vi "LeCroy Wave Series Acquire and Read MyMeasurements.vi"() -> ()   [LabVIEW 2013]
doc: "This example shows how to use autosetup and acquire a waveform on a single channel."
uses:
  <instrlib>/LeCroy Wave Series/Public/Data/Read Waveform Measurement (Px).vi
  <instrlib>/LeCroy Wave Series/LeCroy Wave Series.lvlib
panel:
  out "Status":string
  out "Value":dbl format="%#_6p"
  in  "Parameter (0: P1)":u16(ring) items=["P1", "P2", "P3", "P4", "P5", "P6", "P7", "P8"]
  in  "VISA resource name":refnum<visa-resource-name>
  in  "Timeout (10000 ms)":u32=10000
  # "(c) 2008 - 2012 NATIONAL INSTRUMENTS.  ALL RIGHTS RESERVED."
  # "Directions:\n\n1. Setup the scope to be able to successfully single trigger on a signal applied to the channel selected in the \"Source\" control.\n\n2. On this front panel, enter the VISA Resource name for your scope. (e.g. VICP::123.45.67.8 for TCP/IP, GPIB::5::INSTR for GPIB). Modify the timeout if necessary.\n\n3. Select a parameter to read back\n\n4. Run the VI to trigger the scope and to read back the measurement result."
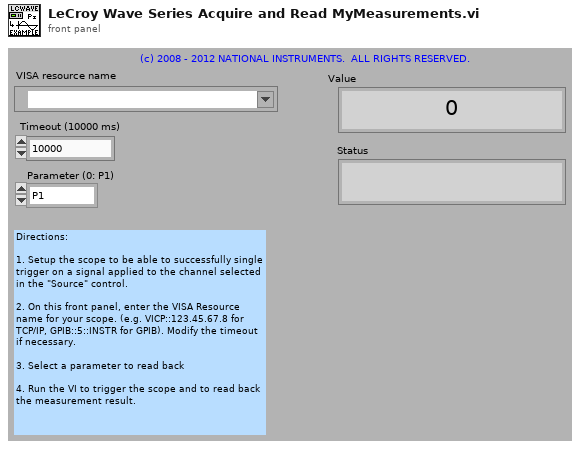
[diagram p1: front panel]
types:
  T1 = enum16{"MyMeasure", "Standard Vertical", "Standard Horizontal"}
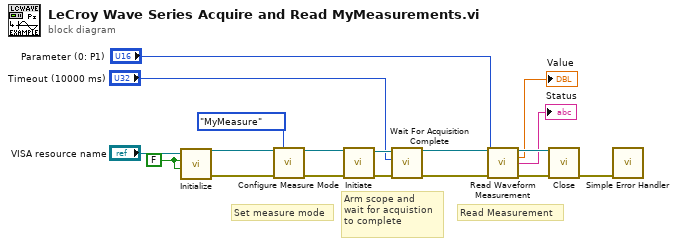
[diagram p0: block diagram]
diagram:
  w14 = FALSE ("ID Query? (T: Yes)")
  # "Arm scope and \nwait for acquistion\nto complete"
  # "Set measure mode"
  # "Read Measurement"
  n1 = call <instrlib>:"Initialize.vi"("Reset? (T: Yes)"=w14, "ID Query? (T: Yes)"=w14, "VISA resource name"="VISA resource name") -> ("error out"=w11:errorcluster, "VISA resource name out"=w13:refnum<visa-resource-name>)  [unwired: 7 in]
  n2 = call <instrlib>:"Configure Measure Mode.vi"("VISA resource name"=w13, "MeasureMode (0=MyMeasure)"=T1."MyMeasure", "error in (no error)"=w11) -> ("VISA resource name out"=w10:refnum<visa-resource-name>, "error out"=w9:errorcluster)  [unwired: 11 in]
  n3 = call <instrlib>:"Initiate.vi"("error in (no error)"=w9, "VISA resource name"=w10) -> ("error out"=w7:errorcluster, "VISA resource name out"=w8:refnum<visa-resource-name>)  [unwired: 8 in]
  n4 = call <instrlib>:"Wait For Acquisition Complete.vi"("error in (no error)"=w7, "Timeout (10000 ms)"="Timeout (10000 ms)", "VISA resource name"=w8) -> ("error out"=w6:errorcluster, "VISA resource name out"=w5:refnum<visa-resource-name>)  [unwired: 6 in, 1 out]
  n5 = call-poly <instrlib>:"Read Waveform Measurement.vi"("VISA resource name"=w5, "Parameter (0: P1)"="Parameter (0: P1)", "error in (no error)"=w6) -> ("VISA resource name out"=w17:refnum<visa-resource-name>, "Value"=→"Value":dbl, "Status"=→"Status":string, "error out"=w16:errorcluster)  [unwired: 9 in]
  n6 = call <instrlib>:"Close.vi"("error in (no error)"=w16, "VISA resource name"=w17) -> ("error out"=w18:errorcluster)  [unwired: 9 in]
  n7 = call <vilib>:"Simple Error Handler.vi"("error in (no error)"=w18) -> ()  [unwired: 4 in, 5 out]
